vi "oax_gsTime Waveform and Speed Profile.vi"() -> ()   [LabVIEW 2017]
doc: "This is Order Analysis Toolkit demo VI."
uses:
  <vilib>/addons/Sound and Vibration/Order Analysis/Utility/SubVIs/oa_Buffer Settings.ctl
  <vilib>/Waveform/WDTOps.llb/WDT Waveform Duration DBL.vi
  <vilib>/addons/Sound and Vibration/Order Analysis/Tach Process/SoundVib_TachProcess.lvlib
  <vilib>/addons/Sound and Vibration/svt_Level/SoundVib_VibrationLevel.lvlib
  <vilib>/addons/Sound and Vibration/Order Analysis/Utility/SoundVib_OAUtility.lvlib
panel:
  in  "STOP":bool
  in  "restart averaging":bool
  out "peak level [EU pk]":dbl=nan format="%.2f"
  out "RMS level [EU rms]":dbl format="%.2f"
  in  "buffer settings":T1={"buffer size"=10.0, "buffer unit"=enum."s"}
  out "speed profile":cluster{"X":dbl[], "Y":dbl[]}(graph)
  out "time waveform":waveform(dbl)(graph)
  in  "Select Data":i32(listbox)
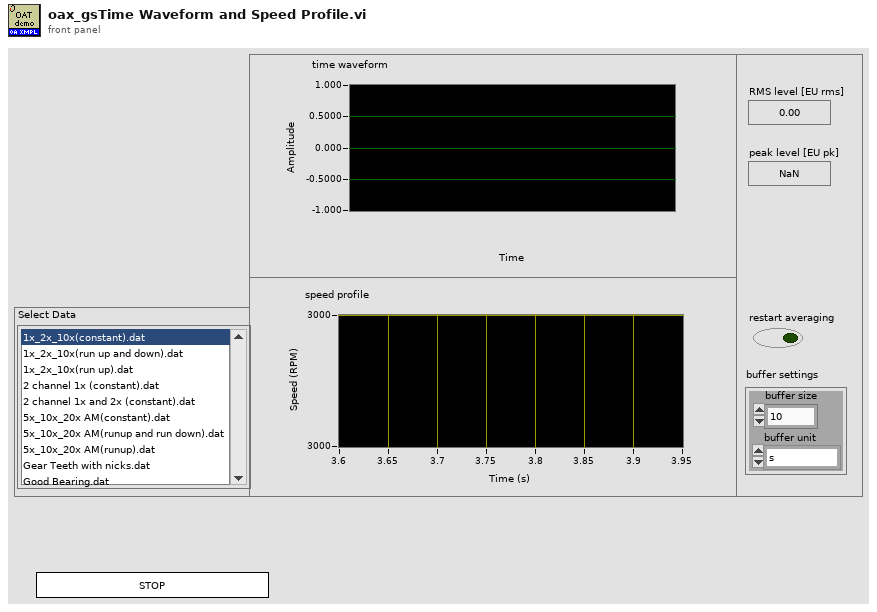
[diagram p1: front panel]
types:
  T1 = typedef "SoundVib_OAUtility.lvlib/oa_Buffer Settings.ctl" = cluster{"buffer size":dbl, "buffer unit":enum16{"s", "revolution", "# of samples"}}
  T2 = typedef "SoundVib_TachProcess.lvlib/speed profile.ctl" = cluster{"time [s]":dbl[], "speed [RPM]":dbl[]}
  T3 = typedef "OAT Position Info.ctl" = cluster{"positions [s]":dbl[], "samples/rev":dbl}
  T4 = cluster{"pulse / rev":i32, "threshold (auto)":dbl, "slope (Rising)":u16}
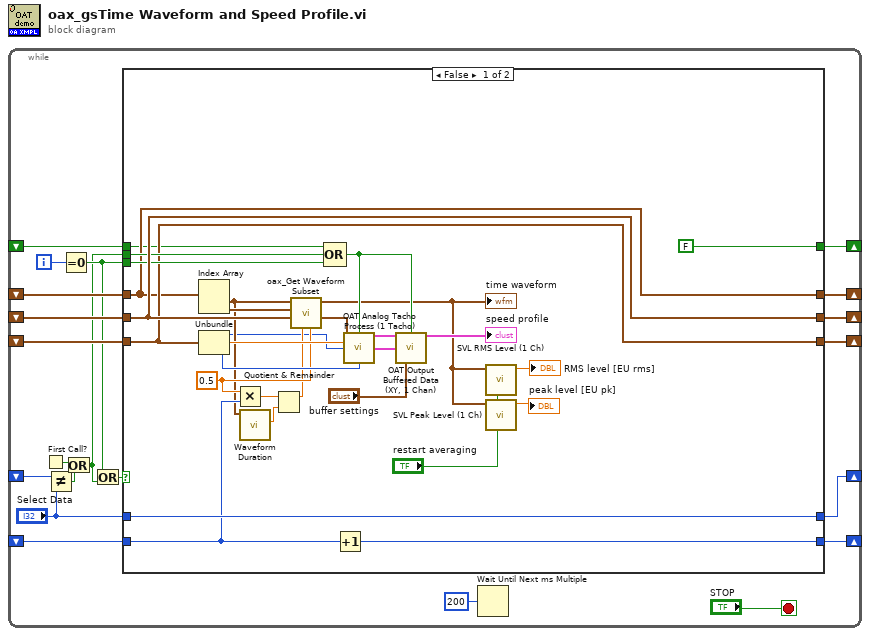
[diagram p0: block diagram]
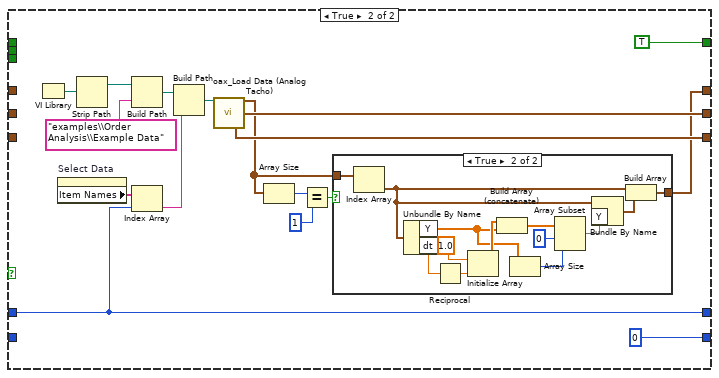
[diagram p2: hidden frame]
diagram:
  n1 = while {
    shift-right: [w18] -> _
    shift-left: _ -> [w19]
    shift-right: [w16] -> _
    shift-left: _ -> [w21]
    shift-right: [w15] -> _
    shift-left: _ -> [w20]
    shift-right: [w14] -> _
    shift-left: _ -> [w13]
    shift-right: [w4] -> _
    shift-left: _ -> [w5]
    shift-right: [w3] -> _
    shift-left: _ -> [w2]
    i -> [w12]
    stop <- "STOP" stop-if-true
    n2 = First Call?() -> (First Call?: T/F=w8:bool)
    n3 = Not Equal?(x=w19, y="Select Data") -> (x != y?=w7:bool)
    n4 = Equal To 0?(x=w12) -> (x = 0?=w11:bool)
    n5 = Or(x=w8, y=w7) -> (x .or. y?=w6:bool)
    n6 = Or(x=w11, y=w6) -> (x .or. y?=w10:bool)
    n7 = case shown="False" w10 {
      tunnel: w21 -> [w32 _]
      tunnel: w20 -> [w48 _]
      tunnel: [w49 w66] -> w18
      tunnel: "Select Data" -> [w49 w66]
      tunnel: [w32 w51] -> w16
      tunnel: [w48 w64] -> w15
      tunnel: [w42 w63] -> w14
      tunnel: w13 -> [w42 _]
      tunnel: w6 -> [w46 _]
      tunnel: w11 -> [w45 _]
      tunnel: w5 -> [w37 _]
      tunnel: [w39 0] -> w4
      tunnel: [FALSE TRUE] -> w3
      tunnel: w2 -> [w22 _]
      frame False {
        w38 = 0.5 ("y")
        n8 = Index Array(array=w32) -> (element #1=w36:waveform(dbl), element #2=w43:waveform(dbl))  [unwired: 2 in]
        n9 = Unbundle(w42) -> ("pulse / rev"=w25:i32, "threshold (auto)"=w41:dbl, "slope (Rising)"=w40:u16)
        n10 = Multiply(x=w38, y=w37) -> (x*y=w34:dbl)
        n11 = call-poly <vilib>:"Waveform Duration.vi"("waveform in"=w36) -> ("duration"=w35:dbl)  [unwired: 8 in, 2 out]
        n12 = Quotient & Remainder(x=w34, y=w35) -> (x-y*floor(x/y)=w33:dbl)  [unwired: 1 out]
        n13 = call <vilib>:"oax_Get Waveform Subset.vi"("duration"=w38, "start index"=w33, "Tach Signal"=w48, "Vibration Signal Y"=w43, "Vibration Signal X"=w36) -> ("Tach Signal out"=w47:waveform(dbl), "Vibration Signal X out"=w23:waveform(dbl))  [unwired: 3 in, 2 out]
        "time waveform" <- w23
        n14 = Compound Arithmetic op=OR(w22, w46, w45) -> (w44:bool)
        n15 = Increment(x=w37) -> (x+1=w39:i32)
        n16 = call <vilib>:"OAT Analog Tacho Process (1 Tacho).vi"("analog tacho signal"=w47, "reset? (F)"=w44, "threshold (auto)"=w41, "pulse/revolution (1)"=w25, "slope (Rising)"=w40) -> ("speed profile"=w50:T2, "speed position info"=w24:T3)  [unwired: 6 in, 3 out]
        n17 = call <vilib>:"OAT Output Buffered Data (XY, 1 Chan).vi"("XY signal"=w50, "reset? (F)"=w44, "position info"=w24, "buffer settings"="buffer settings") -> ("buffered XY signal"=→"speed profile":cluster{"X":dbl[], "Y":dbl[]})  [unwired: 9 in, 2 out]
        n18 = call <vilib>:"SVL RMS Level (1 Ch).vi"("restart averaging (F)"="restart averaging", "scaled signal [EU]"=w23) -> ("RMS level [EU rms]"=→"RMS level [EU rms]":dbl)  [unwired: 7 in, 2 out]
        n19 = call <vilib>:"SVL Peak Level (1 Ch).vi"("restart averaging (F)"="restart averaging", "scaled signal [EU]"=w23) -> ("peak level [EU]"=→"peak level [EU pk]":dbl)  [unwired: 7 in, 2 out]
      }
      frame True {
        n20 = VI Library() -> (path=w59:path)
        n21 = property on="Select Data" class="LstBox (strict)"() -> ("Item Names"=w67:string[])  [unwired: 2 in, 2 out]
        n22 = Strip Path(path=w59) -> (stripped path=w58:path)  [unwired: 1 out]
        n23 = Build Path(base path=w58, name or relative path="examples\\Order Analysis\\Example Data") -> (appended path=w62:path)
        n24 = Index Array(array=w67, index=w66) -> (element=w61:string)
        n25 = Build Path(base path=w62, name or relative path=w61) -> (appended path=w60:path)
        n26 = call <vilib>:"oax_Load Data (Analog Tacho).vi"("Data Path In"=w60) -> ("vibration data"=w52:waveform(dbl)[], "analog tacho signal"=w64:waveform(dbl), "tacho info"=w63:T4)  [unwired: 8 in, 4 out]
        n27 = Array Size(array=w52) -> (size(s)=w55:i32)
        n28 = Equal?(x=w55, y=1) -> (x = y?=w53:bool)
        n29 = case shown="True" w53 {
          tunnel: w52 -> [w68 w81]
          tunnel: [w68 w80] -> w51
          frame False {
          }
          frame True {
            n30 = Index Array(array=w81) -> (element=w79:waveform(dbl))  [unwired: 1 in]
            n31 = Unbundle By Name(w79) -> ("Y"=w71:dbl[], "dt"=w77:dbl)
            n32 = Reciprocal(x=w77) -> (1/x=w69:dbl)
            n33 = Initialize Array(1.0 ("element"), w69) -> (w73:dbl[])
            n34 = Build Array (concatenate)(w73, w71) -> (w75:dbl[])
            n35 = Array Size(array=w71) -> (size(s)=w72:i32)
            n36 = Array Subset(array=w75, index=0, length=w72) -> (w70:dbl[])
            n37 = Bundle By Name(cluster=w79, "Y"=w70) -> (w78:waveform(dbl))
            n38 = Build Array(w79, w78) -> (w80:waveform(dbl)[])
          }
        }
      }
    }
    n39 = Wait Until Next ms Multiple(millisecond multiple=u32 200) -> ()  [unwired: 1 out]
  }
